vi "RollingDice-NoSubVI.vi"() -> ()   [LabVIEW 2018]
panel:
  out "You Win":bool
  out "You Lose":bool
  out "Sum":dbl
  in  "Roll Dice":bool
  out "Dice 2":dbl
  out "Dice 1":dbl
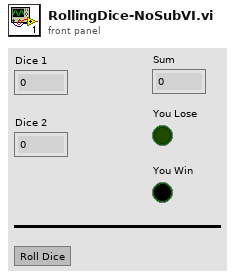
[diagram p1: front panel]
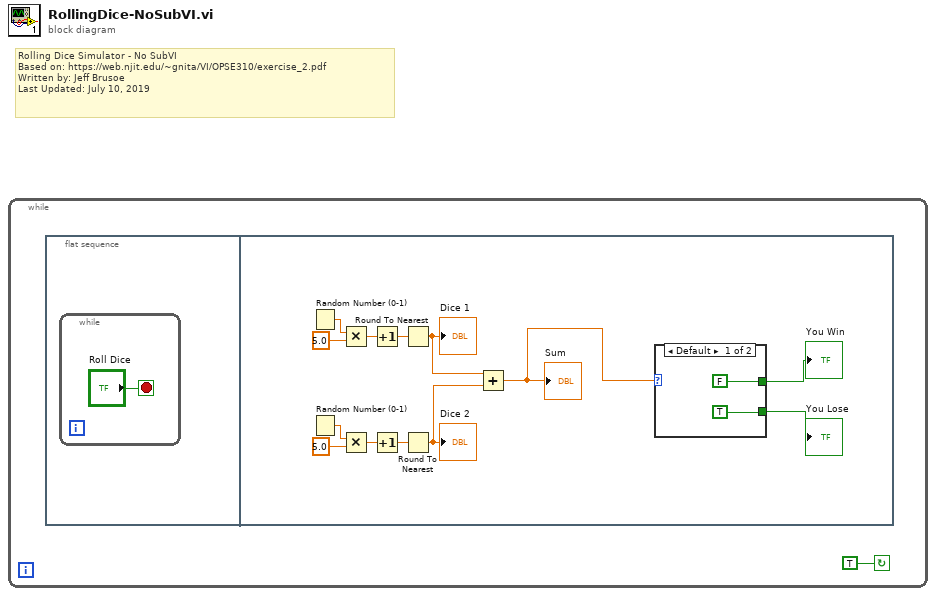
[diagram p0: block diagram]
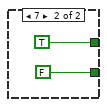
[diagram p2: hidden frame]
diagram:
  # "Rolling Dice Simulator - No SubVI\nBased on: https://web.njit.edu/~gnita/VI/OPSE310/exercise_2.pdf\nWritten by: Jeff Brusoe\nLast Updated: July 10, 2019"
  n1 = while {
    stop <- TRUE continue-if-true
    n2 = flat-sequence {
      frame #0 {
        n3 = while {
          stop <- "Roll Dice" stop-if-true
        }
      }
      frame #1 {
        n4 = Random Number (0-1)() -> (number: 0 to 1=w10:dbl)
        n5 = Random Number (0-1)() -> (number: 0 to 1=w13:dbl)
        n6 = Multiply(x=w10, y=5.0) -> (x*y=w11:dbl)
        n7 = Multiply(x=w13, y=5.0) -> (x*y=w14:dbl)
        n8 = Increment(x=w11) -> (x+1=w12:dbl)
        n9 = Increment(x=w14) -> (x+1=w15:dbl)
        n10 = Round To Nearest(number=w12) -> (nearest integer value=w7:dbl)
        "Dice 1" <- w7
        n11 = Round To Nearest(number=w15) -> (nearest integer value=w6:dbl)
        "Dice 2" <- w6
        n12 = Add(x=w7, y=w6) -> (x+y=w5:dbl)
        "Sum" <- w5
        n13 = case shown="Default" w5 {
          tunnel: [FALSE TRUE] -> w4
          tunnel: [TRUE FALSE] -> w3
          frame Default {
          }
          frame 7 {
          }
        }
        "You Win" <- w4
        "You Lose" <- w3
      }
    }
  }
